vi "main_control Main.vi"() -> ()   [LabVIEW 2024]
doc: "Use this template to build a simple state machine design pattern. Each state executes code and determines which state to transition to."
uses:
  controls/main_control State.ctl
  controls/main_control Data.ctl
  <vilib>/DAQmx/create/channels.llb/DAQmx Create Channel (AI-Voltage-Basic).vi
panel:
  in  "Connect DAQ":bool
  in  "Connect LD Control":bool
  out "Sample taken":bool
  out "Waveform Chart":dbl(graph)
  out "standard deviation":dbl
  out "mean":dbl
  in  "mean iterations":i32
  in  "Stop Sweep":bool
  out "Sweep Running":bool
  in  "Current Step":dbl format="%#_13g"
  in  "Final value (mA)":dbl format="%#_13g"
  in  "Interval (mA)":dbl format="%#_13g"
  in  "Initial value (mA)":dbl format="%#_13g"
  in  "Init Sweep":bool
  out "Steps":dbl format="%#_13g"
  in  "Data Acquisition":bool
  in  "Exit":bool
  in  "CH. AI Input":tag
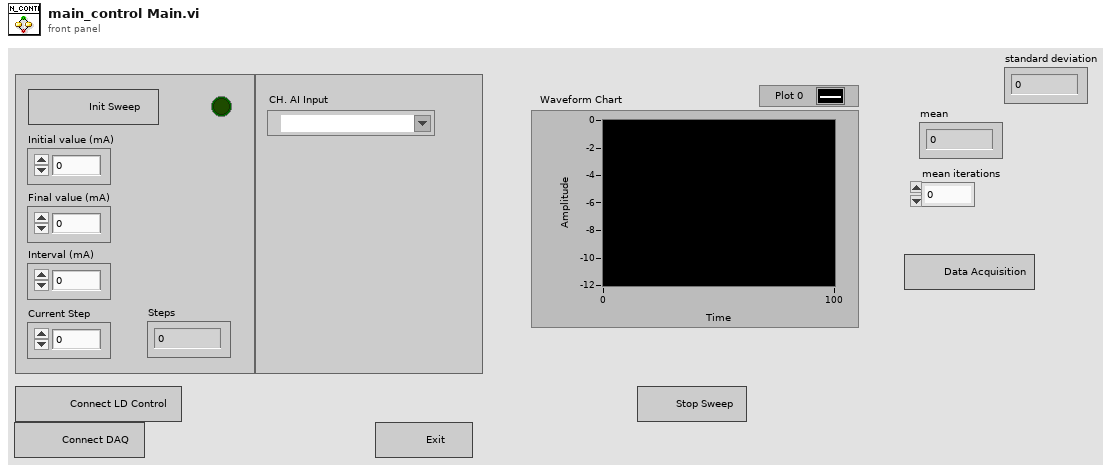
[diagram p1: front panel]
types:
  T1 = cluster{"Steps":refnum<vi>, "Current Step":refnum<vi>, "Final value (mA)":refnum<vi>, "Initial value (mA)":refnum<vi>, "Interval (mA)":refnum<vi>, "Data Acquisition":refnum<vi>, "Init Sweep":refnum<vi>, "Sweep Running":refnum<vi>, "Sample taken":refnum<vi>, "Connect DAQ":refnum<vi>, "Connect LD Control":refnum<vi>}
  T2 = typedef "main_control Data.ctl" = cluster{"Boolean <Replace Me>":bool, "State":string, "Numeric <Replace Me>":dbl}
  T3 = typedef "main_control State.ctl" = enum16{"Initialize", "Connect DAQ", "Connect LD Control", "Wait for Event", "Data Acquisition", "Freq Sweep (Current)", "Exit"}
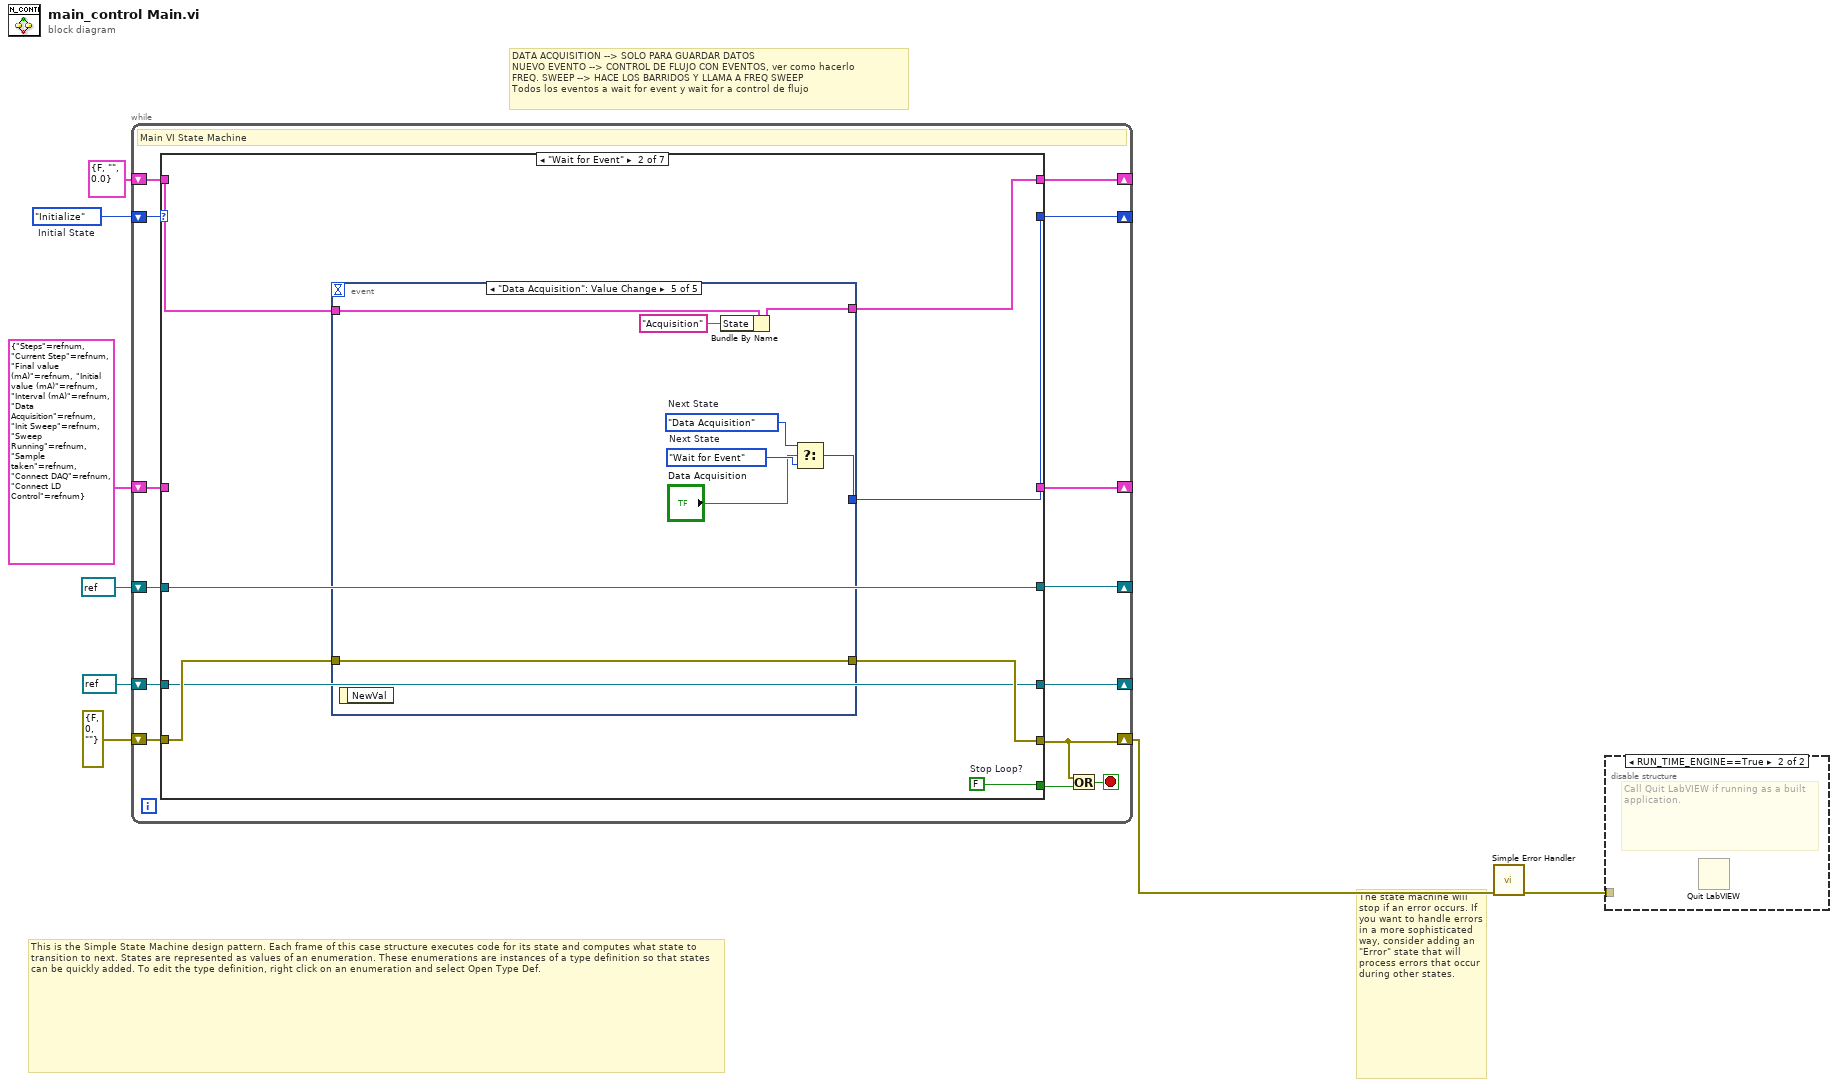
[diagram p0: block diagram]
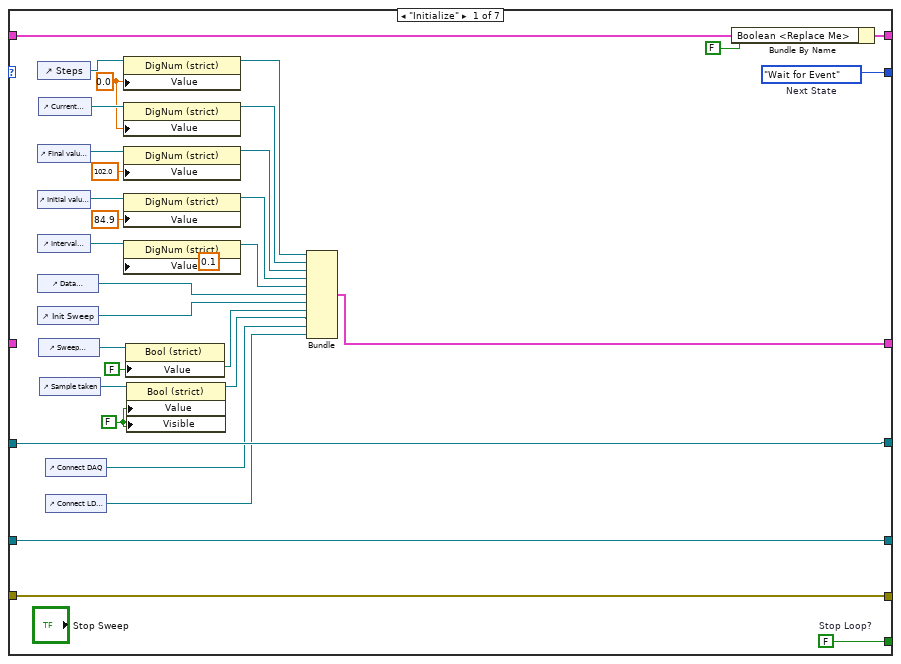
[diagram p3: hidden frame]
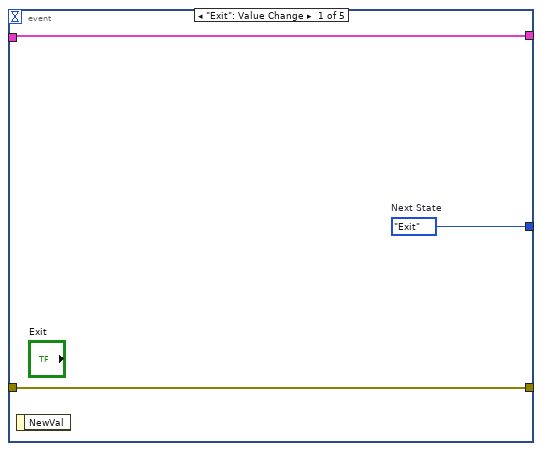
[diagram p4: hidden frame]
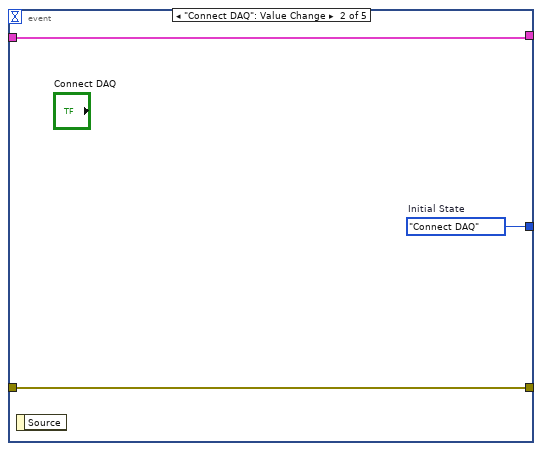
[diagram p5: hidden frame]
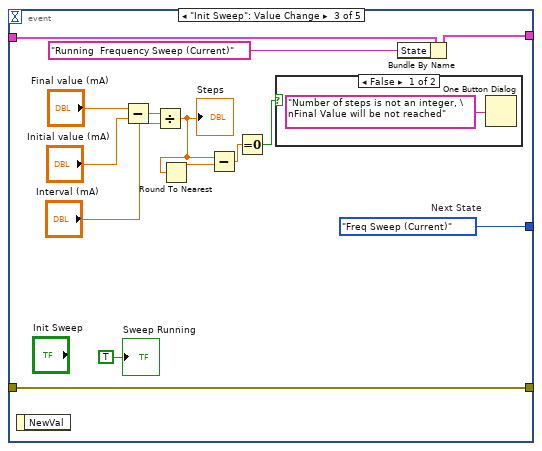
[diagram p6: hidden frame]
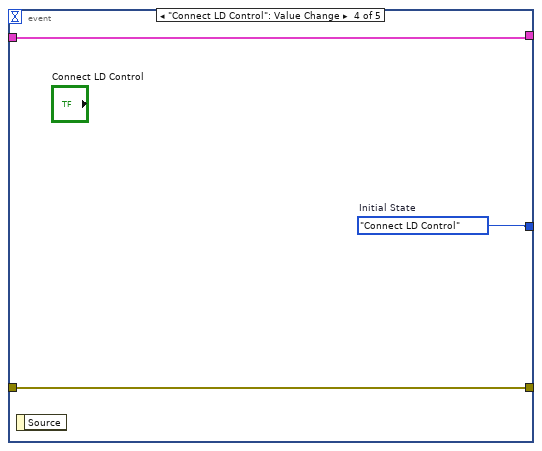
[diagram p8: hidden frame]
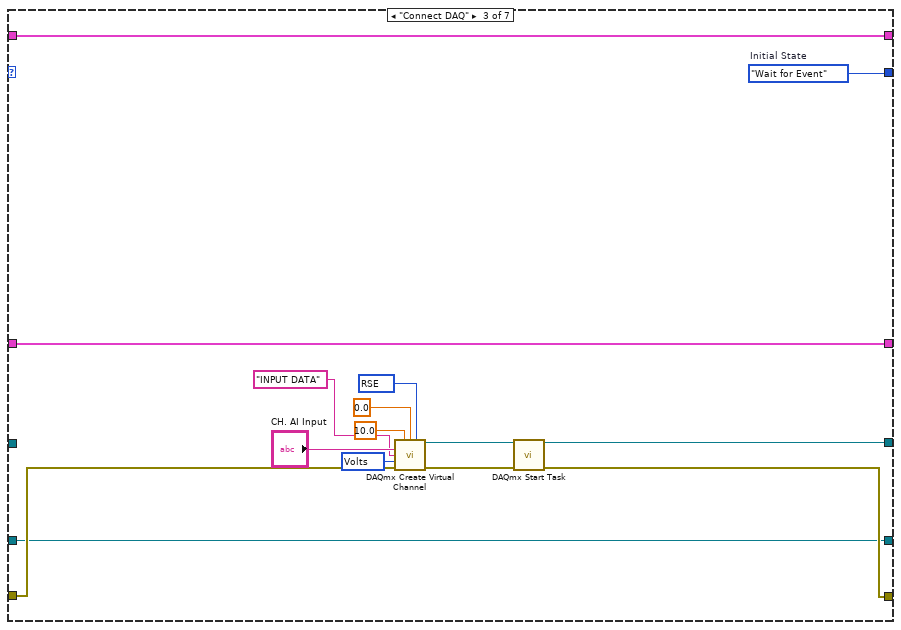
[diagram p9: hidden frame]
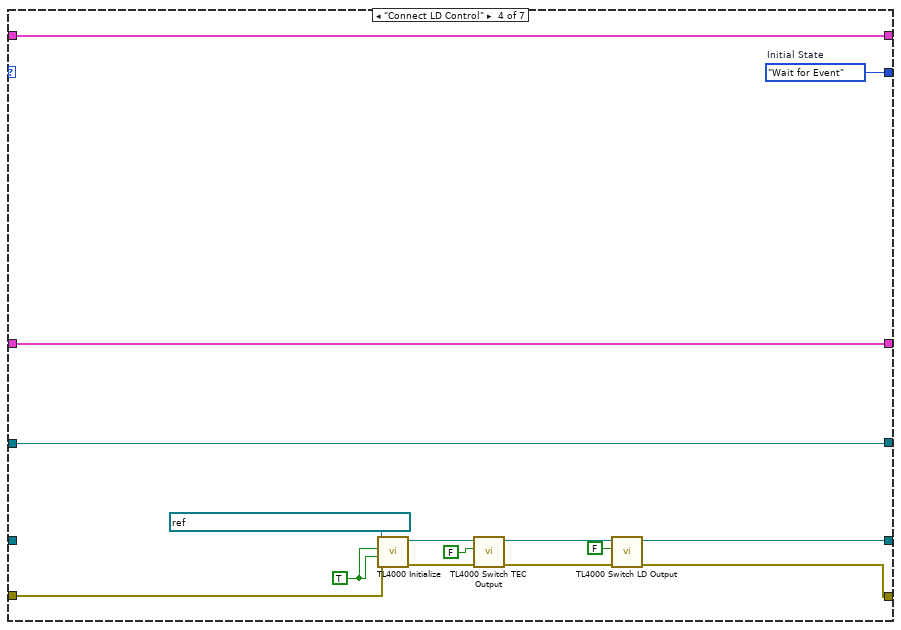
[diagram p10: hidden frame]
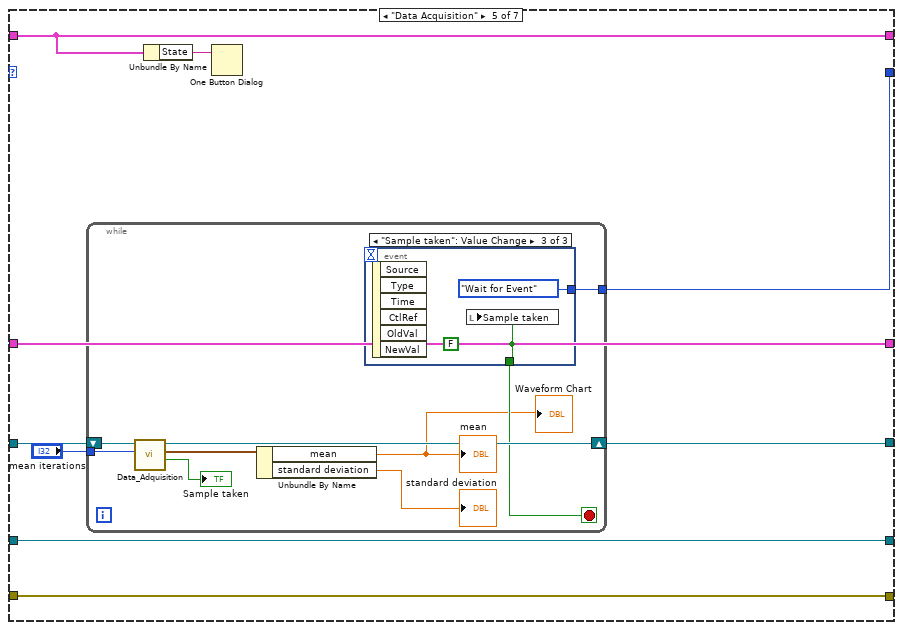
[diagram p11: hidden frame]
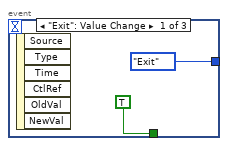
[diagram p12: hidden frame]
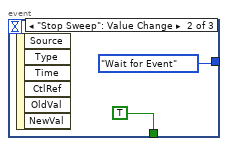
[diagram p13: hidden frame]
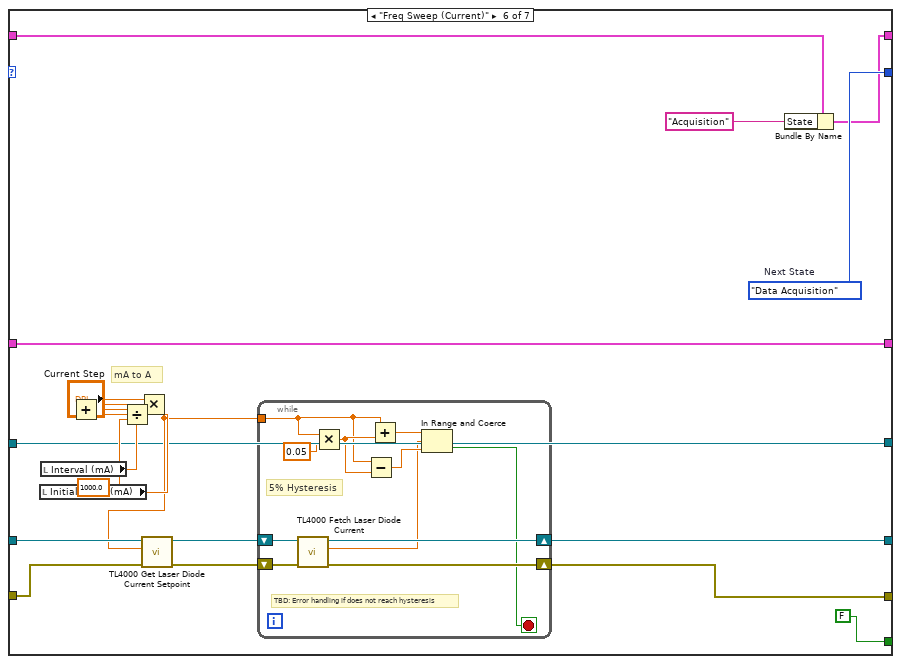
[diagram p14: hidden frame]
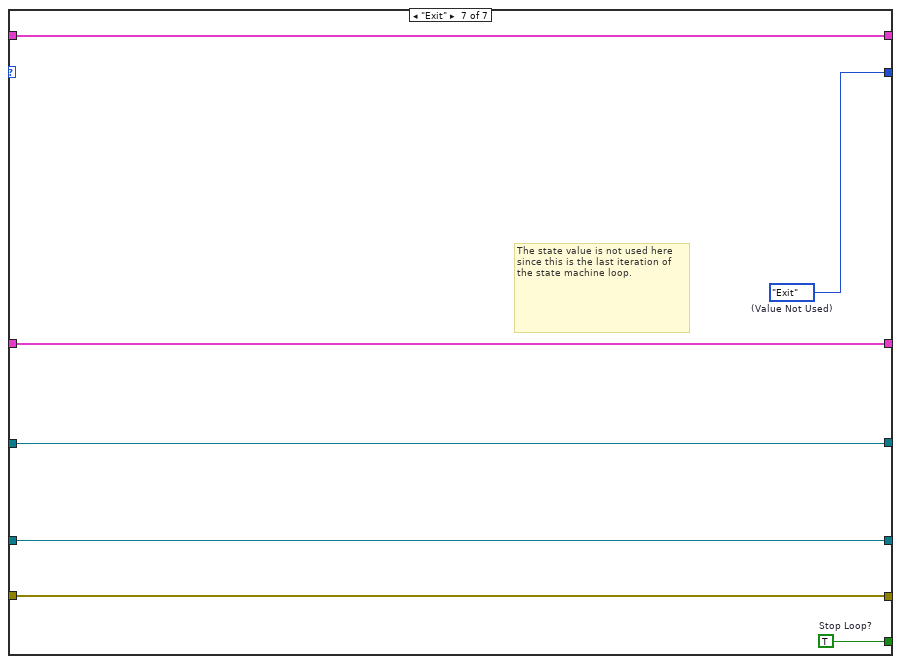
[diagram p15: hidden frame]
diagram:
  w8 = main_control_State."Initialize"  # Initial State
  # "DATA ACQUISITION --> SOLO PARA GUARDAR DATOS\nNUEVO EVENTO --> CONTROL DE FLUJO CON EVENTOS, ver como hacerlo\nFREQ. SWEEP --> HACE LOS BARRIDOS Y LLAMA A FREQ SWEEP\nTodos los eventos a wait for event y wait for a control de flujo"
  # "The state machine will stop if an error occurs. If you want to handle errors in a more sophisticated way, consider adding an \"Error\" state that will process errors that occur during other states."
  # "This is the Simple State Machine design pattern. Each frame of this case structure executes code for its state and computes what state to transition to next. States are represented as values of an enumeration. These enumerations are instances of a type definition so that states can be quickly added. To edit the type definition, right click on an enumeration and select Open Type Def."
  n1 = while {
    shift-right: [w21] -> _
    shift-left: w8 -> [w22]
    shift-right: [w19] -> _
    shift-left: T2 {"Boolean <Replace Me>"=FALSE, "State"="", "Numeric <Replace Me>"=0.0} ("Data") -> [w20]
    shift-right: [w16] -> _
    shift-left: refnum<visa-resource-name> refnum ("instrument handle out") -> [w13]
    shift-right: [w15] -> w3
    shift-left: errorcluster {"status"=FALSE, "code"=0, "source"=""} ("error out") -> [w14]
    shift-right: [w11] -> _
    shift-left: T1 {"Steps"=refnum, "Current Step"=refnum, "Final value (mA)"=refnum, "Initial value (mA)"=refnum, "Interval (mA)"=refnum, "Data Acquisition"=refnum, "Init Sweep"=refnum, "Sweep Running"=refnum, "Sample taken"=refnum, "Connect DAQ"=refnum, "Connect LD Control"=refnum} -> [w12]
    shift-right: [w10] -> _
    shift-left: refnum<k21> refnum ("task out") -> [w9]
    stop <- w17 stop-if-true
    # "Main VI State Machine"
    n2 = case shown="\"Wait for Event\"" w22 {
      tunnel: [w55 w63 w96 w112 w126 w169 w187] -> w21
      tunnel: [w54 w62 _ _ _ FALSE ("Stop Loop?") w185] -> w18
      tunnel: w20 -> [w53 w61 w110 w125 w134 w152 w186]
      tunnel: [w52 w60 w110 w125 w134 w153 w186] -> w19
      tunnel: [w27 w57 w97 w117 w131 w156 w183] -> w16
      tunnel: [w26 w58 w99 w116 w130 w157 w182] -> w15
      tunnel: w14 -> [w26 w59 w100 w115 w130 w166 w182]
      tunnel: w13 -> [w27 w57 w97 _ w131 w167 w183]
      tunnel: [w34 _ w98 w113 w132 w151 w184] -> w11
      tunnel: w12 -> [_ _ w98 w113 w132 w151 w184]
      tunnel: [w25 w56 w101 w114 w128 w150 w181] -> w10
      tunnel: w9 -> [w25 w56 _ w114 w129 w150 w181]
      frame "Initialize" {
        w29 = FALSE ("Value")
        w42 = 0.0
        w54 = FALSE  # Stop Loop?
        w55 = main_control_State."Wait for Event"  # Next State
        # "Initialize - Initialize the application."
        n3 = control-ref of="Steps"() -> (w50:refnum<vi>)
        n4 = control-ref of="Final value (mA)"() -> (w49:refnum<vi>)
        n5 = control-ref of="Initial value (mA)"() -> (w48:refnum<vi>)
        n6 = control-ref of="Interval (mA)"() -> (w47:refnum<vi>)
        n7 = control-ref of="Data Acquisition"() -> (w36:refnum<vi>)
        n8 = control-ref of="Init Sweep"() -> (w35:refnum<vi>)
        n9 = control-ref of="Current Step"() -> (w43:refnum<vi>)
        n10 = control-ref of="Sweep Running"() -> (w33:refnum<vi>)
        n11 = control-ref of="Sample taken"() -> (w30:refnum<vi>)
        n12 = control-ref of="Connect DAQ"() -> (w23:refnum<vi>)
        n13 = control-ref of="Connect LD Control"() -> (w24:refnum<vi>)
        n14 = property class="DigNum (strict)"(reference=w50, "Value"=w42) -> (reference out=w41:refnum<vi>)  [unwired: 1 in, 1 out]
        n15 = property class="DigNum (strict)"(reference=w43, "Value"=w42) -> (reference out=w40:refnum<vi>)  [unwired: 1 in, 1 out]
        n16 = property class="DigNum (strict)"(reference=w49, "Value"=102.0) -> (reference out=w39:refnum<vi>)  [unwired: 1 in, 1 out]
        n17 = property class="DigNum (strict)"(reference=w48, "Value"=84.9) -> (reference out=w38:refnum<vi>)  [unwired: 1 in, 1 out]
        n18 = property class="DigNum (strict)"(reference=w47, "Value"=0.1) -> (reference out=w37:refnum<vi>)  [unwired: 1 in, 1 out]
        n19 = property class="Bool (strict)"(reference=w33, "Value"=FALSE) -> (reference out=w31:refnum<vi>)  [unwired: 1 in, 1 out]
        n20 = property class="Bool (strict)"(reference=w30, "Value"=w29, "Visible"=w29) -> (reference out=w28:refnum<vi>)  [unwired: 1 in, 1 out]
        n21 = Bundle("Steps"=w41, "Current Step"=w40, "Final value (mA)"=w39, "Initial value (mA)"=w38, "Interval (mA)"=w37, "Data Acquisition"=w36, "Init Sweep"=w35, "Sweep Running"=w31, "Sample taken"=w28, "Connect DAQ"=w23, "Connect LD Control"=w24) -> (w34:T1)  [unwired: 1 in]
        n22 = Bundle By Name(cluster=w53, "Boolean <Replace Me>"=FALSE ("Replace_Me_Boolean")) -> (w52:T2)
      }
      frame "Wait for Event" {
        w62 = FALSE  # Stop Loop?
        # "Wait for Event - Use an Event Structure to monitor the user interface for events that run different states of the state machine."
        n23 = event shown="[4] \"Data Acquisition\": Value Change" {
          selector: _ -> [_ _ _ _ _]
          dyn-events: _ -> [_ _ _ _ _]
          timeout: _ -> [_ _ _ _ _]
          tunnel: [w66 w67 w83 w85 w91] -> w63
          tunnel: w61 -> [w65 w69 w82 w87 w95]
          tunnel: [w65 w69 w81 w87 w94] -> w60
          tunnel: w59 -> [w64 w68 w79 w86 w92]
          tunnel: [w64 w68 w79 w86 w92] -> w58
          event "Exit": Value Change {
            w66 = main_control_State."Exit"  # Next State
            n24 = event-data() -> ()  [unwired: 1 in, 1 out]
          }
          event "Connect DAQ": Value Change {
            w67 = main_control_State."Connect DAQ"  # Initial State
            n25 = event-data() -> ()  [unwired: 1 in, 1 out]
          }
          event "Init Sweep": Value Change {
            w83 = main_control_State."Freq Sweep (Current)"  # Next State
            n26 = event-data() -> ()  [unwired: 1 in, 1 out]
            n27 = Subtract(x="Final value (mA)", y="Initial value (mA)") -> (x-y=w77:dbl)
            n28 = Divide(x=w77, y="Interval (mA)") -> (x/y=w72:dbl)
            "Steps" <- w72
            n29 = Round To Nearest(number=w72) -> (nearest integer value=w73:dbl)
            n30 = Subtract(x=w72, y=w73) -> (x-y=w71:dbl)
            n31 = Equal To 0?(x=w71) -> (x = 0?=w70:bool)
            n32 = case shown="False" w70 {
              frame False {
                n33 = One Button Dialog(message="Number of steps is not an integer, \nFinal Value will be not reached") -> ()  [unwired: 1 in, 1 out]
              }
              frame True {
              }
            }
            n34 = Bundle By Name(cluster=w82, "State"="Running  Frequency Sweep (Current)" ("Running User State 1")) -> (w81:T2)
            "Sweep Running" <- TRUE ("Sweep Running")
          }
          event "Connect LD Control": Value Change {
            w85 = main_control_State."Connect LD Control"  # Initial State
            n35 = event-data() -> ()  [unwired: 1 in, 1 out]
          }
          event "Data Acquisition": Value Change {
            w89 = main_control_State."Wait for Event"  # Next State
            w90 = main_control_State."Data Acquisition"  # Next State
            n36 = event-data() -> ()  [unwired: 1 in, 1 out]
            n37 = Bundle By Name(cluster=w95, "State"="Acquisition" ("Running User State 2")) -> (w94:T2)
            n38 = Select(t=w90, s="Data Acquisition", f=w89) -> (s? t:f=w91:T3)
          }
        }
      }
      frame "Connect DAQ" {
        w96 = main_control_State."Wait for Event"  # Initial State
        w102 = 10348 items=["Volts"=10348, "From Custom Scale"=10065] ("units")
        w104 = 10083 items=["Default"=-1, "RSE"=10083, "NRSE"=10078, "Differential"=10106, "Pseudodifferential"=12529] ("input terminal configuration")
        n39 = call-poly <vilib>:"DAQmx Create Virtual Channel.vi"("maximum value"=10.0, "minimum value"=0.0, "input terminal configuration"=w104, "physical channels"="CH. AI Input", "name to assign"="INPUT DATA", "units"=w102, "error in"=w100) -> ("task out"=w107:refnum<k21>, "error out"=w108:errorcluster)  [unwired: 7 in]
        n40 = call <vilib>:"DAQmx Start Task.vi"("task/channels in"=w107, "error in"=w108) -> ("task out"=w101:refnum<k21>, "error out"=w99:errorcluster)  [unwired: 12 in]
      }
      frame "Connect LD Control" {
        w112 = main_control_State."Wait for Event"  # Initial State
        w118 = TRUE
        n41 = call <instrlib>:"TL4000 Initialize.vi"("error in (no error)"=w115, "Reset Device (Reset Device)"=w118, "ID Query (Do Query)"=w118, "resource name"=refnum<visa-resource-name> "USB0::0x1313::0x804F::M00287955::INSTR") -> ("error out"=w124:errorcluster, "instrument handle out"=w123:refnum<visa-resource-name>)  [unwired: 6 in]
        n42 = call <instrlib>:"TL4000 Switch TEC Output.vi"("error in (no error)"=w124, "TEC Output (Off)"=FALSE, "instrument handle"=w123) -> ("error out"=w121:errorcluster, "instrument handle out"=w122:refnum<visa-resource-name>)  [unwired: 7 in]
        n43 = call <instrlib>:"TL4000 Switch LD Output.vi"("error in (no error)"=w121, "LD Output (Off)"=FALSE, "instrument handle"=w122) -> ("error out"=w116:errorcluster, "instrument handle out"=w117:refnum<visa-resource-name>)  [unwired: 7 in]
      }
      frame "Data Acquisition" {
        # "User State 1 - Replace this state with functionality for your own application."
        n44 = while {
          tunnel: "mean iterations" -> [w141]
          shift-right: [w142] -> w128
          shift-left: w129 -> [w143]
          tunnel: [w136] -> w126
          stop <- w138 stop-if-true
          n45 = call "Data_Adquisition.vi"("Mean Iterations"=w141, "task in"=w143) -> ("Sample taken"=→"Sample taken":bool, "mean and std"=w140:cluster{"mean":dbl, "standard deviation":dbl}, "task out"=w142:refnum<k21>)  [unwired: 4 in, 1 out]
          n46 = Unbundle By Name(w140) -> ("mean"=→"mean" →"Waveform Chart":dbl, "standard deviation"=→"standard deviation":dbl)
          n47 = event shown="[2] \"Sample taken\": Value Change" {
            selector: _ -> [_ _ _]
            dyn-events: _ -> [_ _ _]
            timeout: _ -> [_ _ _]
            tunnel: [TRUE ("s") TRUE ("s") w149] -> w138
            tunnel: [main_control_State."Exit" ("Next State") main_control_State."Wait for Event" ("Next State") main_control_State."Wait for Event"] -> w136
            event "Exit": Value Change {
              n48 = event-data() -> ()  [unwired: 1 in, 6 out]
            }
            event "Stop Sweep": Value Change {
              n49 = event-data() -> ()  [unwired: 1 in, 6 out]
            }
            event "Sample taken": Value Change {
              w149 = FALSE
              n50 = event-data() -> ()  [unwired: 1 in, 6 out]
              n51 = local write "Sample taken"(w149) -> ()
            }
          }
        }
        n52 = Unbundle By Name(w134) -> ("State"=w133:string)
        n53 = One Button Dialog(message=w133) -> ()  [unwired: 1 in, 1 out]
      }
      frame "Freq Sweep (Current)" {
        w169 = main_control_State."Data Acquisition"  # Next State
        # "mA to A"
        # "User State 2 - Replace this state with functionality for your own application."
        n54 = local read "Initial value (mA)"() -> (w163:dbl)
        n55 = local read "Interval (mA)"() -> (w164:dbl)
        n56 = Multiply(x="Current Step", y=w164) -> (x*y=w162:dbl)
        n57 = Add(x=w162, y=w163) -> (x+y=w160:dbl)
        n58 = Divide(x=w160, y=1000.0) -> (x/y=w155:dbl)
        n59 = call <instrlib>:"TL4000 Get Laser Diode Current Setpoint.vi"("error in (no error)"=w166, "Attribute (Set value)"=w155, "instrument handle"=w167) -> ("error out"=w158:errorcluster, "instrument handle out"=w159:refnum<visa-resource-name>)  [unwired: 6 in, 1 out]
        n60 = while {
          shift-right: [w177] -> w156
          shift-left: w159 -> [w180]
          shift-right: [w178] -> w157
          shift-left: w158 -> [w179]
          tunnel: w155 -> [w172]
          stop <- w170 stop-if-true
          # "TBD: Error handling if does not reach hysteresis"
          # "5% Hysteresis"
          n61 = call <instrlib>:"TL4000 Fetch Laser Diode Current.vi"("error in (no error)"=w179, "instrument handle"=w180) -> ("error out"=w178:errorcluster, "Current"=w171:dbl, "instrument handle out"=w177:refnum<visa-resource-name>)  [unwired: 7 in]
          n62 = Multiply(x=w172, y=0.05) -> (x*y=w174:dbl)
          n63 = Subtract(x=w172, y=w174) -> (x-y=w173:dbl)
          n64 = Add(x=w172, y=w174) -> (x+y=w175:dbl)
          n65 = In Range and Coerce(upper limit=w175, x=w171, lower limit=w173) -> (In Range?=w170:bool)  [unwired: 1 out]
        }
        n66 = Bundle By Name(cluster=w152, "State"="Acquisition" ("Running User State 2")) -> (w153:T2)
      }
      frame "Exit" {
        w185 = TRUE  # Stop Loop?
        w187 = main_control_State."Exit"  # (Value Not Used)
        # "The state value is not used here since this is the last iteration of the state machine loop."
        # "Exit - Exit the application."
      }
    }
    n67 = Or(x=w15, y=w18) -> (x .or. y?=w17:bool)
  }
  n68 = call <vilib>:"Simple Error Handler.vi"("error in (no error)"=w3) -> ("error out"=w6:errorcluster)  [unwired: 4 in, 4 out]
  n69 = disable-structure shown="RUN_TIME_ENGINE==True" {
    disable-tunnel: w6 -> [_ _]
    frame condition #0 (active) {
    }
    frame condition #1 {
      # "Call Quit LabVIEW if running as a built application."
      n70 = Quit LabVIEW() -> ()  [unwired: 1 in]
    }
  }
